vi "Wire Refnum To BBN.vi"(6 "Label.Text":string, 8 "error in":errorcluster, 9 "Created RefNum":refnum<vi>, 10 "VI in":refnum<vi>) -> ()   [LabVIEW 2021, in "_Control To Private Data.lvlib"]
uses:
  _Control To Private Data.lvlib
  <vilib>/Utility/traverseref.llb/TRef TravTarget.ctl
  <vilib>/Utility/traverseref.llb/VI Scripting - Traverse.lvlib
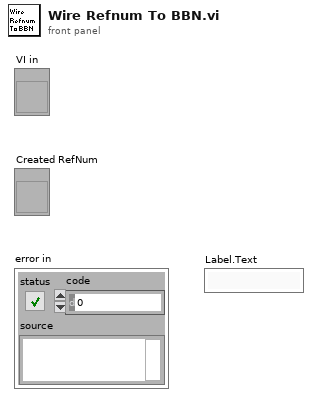
[diagram p1: front panel]
types:
  T1 = typedef "TRef TravTarget.ctl" = enum16{"FP", "BD", "Other"}
  T2 = enum32{"Top Edges", "Vertical Centers", "Bottom Edges", "Vertical Gap", "Vertical Compress", "Left Edges", "Horizontal Centers", "Right Edges", "Horizontal Gap", "Horizontal Compress"}
  T3 = enum32{"Top Edges", "Vertical Centers", "Bottom Edges", "Left Edges", "Horizontal Centers", "Right Edges"}
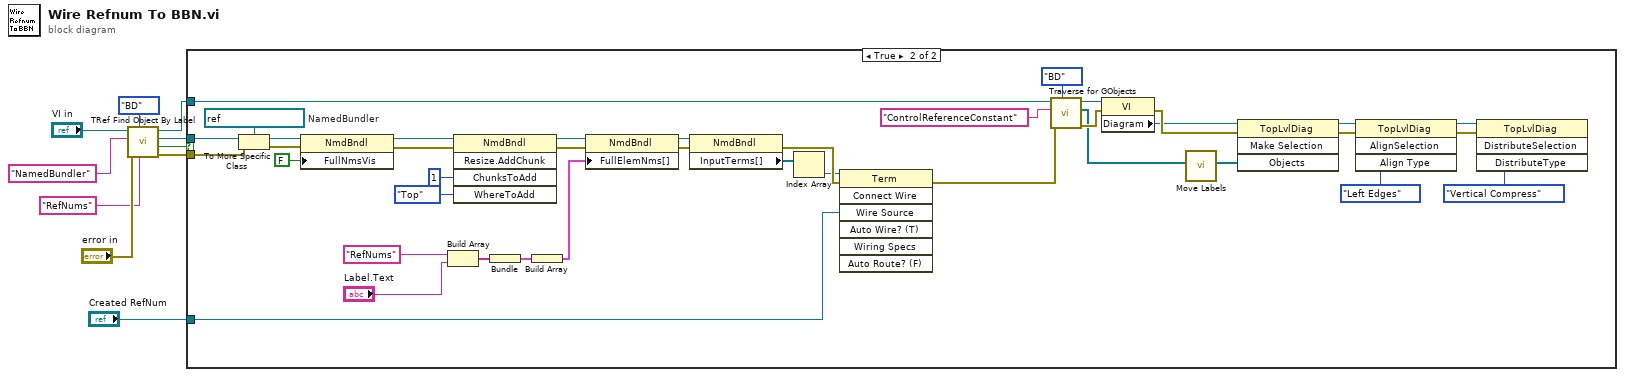
[diagram p0: block diagram]
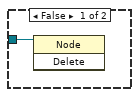
[diagram p2: hidden frame]
diagram:
  n1 = call <vilib>:"TRef Find Object By Label.vi"("Label"="RefNums" ("Label.Text"), "Traverse Target"=TRef_TravTarget."BD", "error in (no error)"="error in", "Class Name"="NamedBundler", "VI Ref"="VI in") -> ("error out"=w9:errorcluster, "Found?"=w4:bool, "Found Obj Ref"=w3:refnum<vi>, "dup VI Ref"=w6:refnum<vi>)  [unwired: 3 in]
  n2 = case shown="True" w4 {
    tunnel: w3 -> [_ w40]
    tunnel: "Created RefNum" -> [w11 w27]
    tunnel: w6 -> [_ w21]
    tunnel: w9 -> [_ w50]
    frame False {
      n3 = invoke class="Node" method="Delete"(reference=w11) -> ()  [unwired: 2 in, 3 out]
    }
    frame True {
      w39 = refnum<vi> refnum  # NamedBundler
      n4 = To More Specific Class(target class=w39, reference=w40, error in=w50) -> (specific class reference=w38:refnum<vi>, error out=w49:errorcluster)
      n5 = property class="NmdBndl"(reference=w38, error in=w49, "FullNmsVis"=FALSE ("Full Names Visible?")) -> (reference out=w34:refnum<vi>, error out=w48:errorcluster)
      n6 = Build Array("RefNums" ("Label.Text"), "Label.Text") -> (w32:string[])
      n7 = invoke class="NmdBndl" method="Resize.AddChunk"(reference=w34, error in=w48, "ChunksToAdd"=u8 1 ("Chunks To Add"), "WhereToAdd"=enum8{"Bottom", "Top"}."Top" ("Where To Add")) -> (reference out=w17:refnum<vi>, error out=w47:errorcluster)  [unwired: 1 in, 3 out]
      n8 = Bundle(w32) -> (w31:cluster{string[]})  [unwired: 1 in]
      n9 = Build Array(w31) -> (w30:cluster{string[]}[])
      n10 = property class="NmdBndl"(reference=w17, error in=w47, "FullElemNms[]"=w30) -> (reference out=w29:refnum<vi>, error out=w46:errorcluster)
      n11 = property class="NmdBndl"(reference=w29, error in=w46) -> (error out=w45:errorcluster, "InputTerms[]"=w33:refnum<vi>[])  [unwired: 1 out]
      n12 = Index Array(array=w33) -> (element=w28:refnum<vi>)  [unwired: 1 in]
      n13 = invoke class="Term" method="Connect Wire"(reference=w28, error in=w45, "Wire Source"=w27) -> (error out=w12:errorcluster)  [unwired: 4 in, 6 out]
      n14 = call <vilib>:"Traverse for GObjects.vi"("Traverse Target"=TRef_TravTarget."BD", "error in (no error)"=w12, "Class Name"="ControlReferenceConstant", "VI Refnum"=w21) -> ("error out"=w44:errorcluster, "References"=w16:refnum<vi>[], "dup VI Refnum"=w19:refnum<vi>)  [unwired: 4 in, 1 out]
      n15 = property class="VI"(reference=w19, error in=w44) -> (error out=w43:errorcluster, "Diagram"=w18:refnum<vi>)  [unwired: 1 out]
      n16 = call "Move Labels.vi"("Objects"=w16) -> ("Objects dup"=w15:refnum<vi>[])  [unwired: 10 in]
      n17 = invoke on="Invoke Node" class="TopLvlDiag" method="Make Selection"(reference=w18, error in=w43, "Objects"=w15) -> (reference out=w20:refnum<vi>, error out=w42:errorcluster)  [unwired: 1 in, 2 out]
      n18 = invoke on="Invoke Node" class="TopLvlDiag" method="AlignSelection"(reference=w20, error in=w42, "Align Type"=T3."Left Edges") -> (reference out=w25:refnum<vi>, error out=w41:errorcluster)  [unwired: 1 in, 2 out]
      n19 = invoke on="Invoke Node" class="TopLvlDiag" method="DistributeSelection"(reference=w25, error in=w41, "DistributeType"=T2."Vertical Compress") -> ()  [unwired: 1 in, 4 out]
    }
  }
